vi "LSX Set Sm Hdi Button.vi"(8 "error in (no error)":errorcluster, 9 "pcFunction":string, 10 "lButtonNr":i32, 11 "lLSID":i32) -> (0 "error out":errorcluster, 1 "pcFunction out":string, 3 "function return":i32)   [LabVIEW 2018, in "Tango.lvlib"]
doc: "TANGOAPI int TANGOCALL LSX_SetSmHdiButton (int lLSID, int lButtonNr, char *pcFunction);"
uses:
  <userlib>/Tango/Tango.lvlib
  <userlib>/Tango/Tango_DLL.dll
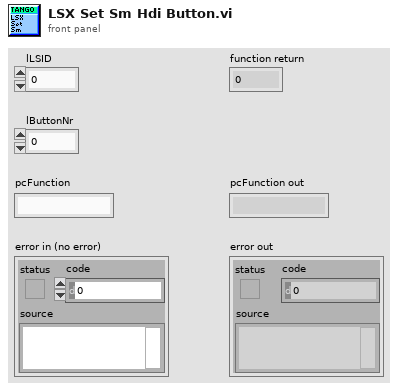
[diagram p1: front panel]
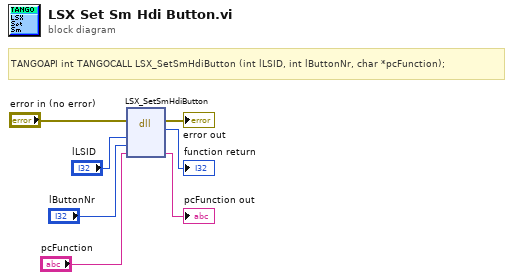
[diagram p0: block diagram]
diagram:
  # "TANGOAPI int TANGOCALL LSX_SetSmHdiButton (int lLSID, int lButtonNr, char *pcFunction);"
  n1 = dll-call lib="C:/Program Files (x86)/National Instruments/LabVIEW 2018/user.lib/Tango/Tango_DLL.*" fn="LSX_SetSmHdiButton"(error in="error in (no error)", "lLSID"="lLSID", "lButtonNr"="lButtonNr", "pcFunction"="pcFunction") -> (error out=→"error out":errorcluster, →"function return":i32, "pcFunction"=→"pcFunction out":string)  [unwired: 4 in, 1 out]
